vi "Validate Endpoint Configuration Reference.vi"(8 "error in":errorcluster, 11 "endpoint configuration in":T1 format="%.0x") -> (0 "error out":errorcluster, 3 "endpoint configuration out":T1 format="%.0x")   [LabVIEW 2017, in "NI-SWITCH Scripting.lvlib"]
uses:
  NI-SWITCH Scripting.lvlib
  <vilib>/NI Veristand/Custom Device API/Custom Device Item Ref.ctl
  SLSC Scripting Constants.vi
  <vilib>/NI VeriStand/Custom Device API/Custom Device API.lvlib
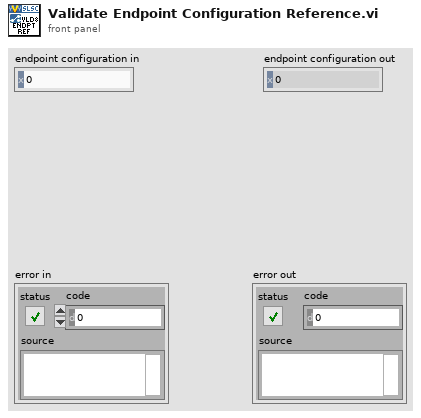
[diagram p1: front panel]
types:
  T1 = typedef "Custom Device API.lvlib/Custom Device Item Ref.ctl" = u64
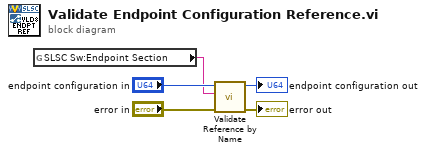
[diagram p0: block diagram]
diagram:
  n1 = global read "SLSC Scripting Constants.vi" "SLSC Sw:Endpoint Section"() -> (w1:string)
  n2 = call "Validate Reference by Name.vi"("error in"="error in", "name"=w1, "slsc switch item in"="endpoint configuration in") -> ("error out"=→"error out":errorcluster, "slsc switch item out"=→"endpoint configuration out":T1)  [unwired: 7 in]
